vi "SetColorState.vi"(8 "error in (no error)":errorcluster, 10 "ColorStateIn":T1, 11 "Boolean in":refnum<vi>) -> (0 "error out":errorcluster, 2 "ColorStateOut":T1)   [LabVIEW 2016]
uses:
  controls/ColorStates.ctl
  controls/RT-Variables.lvlib
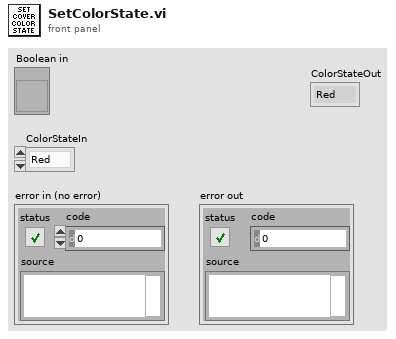
[diagram p1: front panel]
types:
  T1 = typedef "RT-Variables.lvlib/ColorStates.ctl" = enum16{"Red", "Yellow", "Green"}
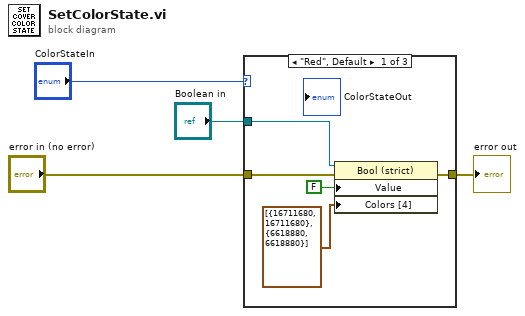
[diagram p0: block diagram]
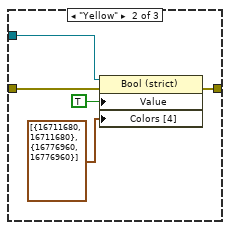
[diagram p2: hidden frame]
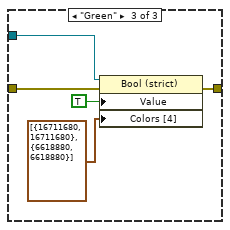
[diagram p3: hidden frame]
diagram:
  n1 = case shown="\"Red\", Default" "ColorStateIn" {
    tunnel: "Boolean in" -> [w7 w12 w17]
    tunnel: "error in (no error)" -> [w6 w11 w15]
    tunnel: [w5 w10 w16] -> w4
    frame "Red", Default {
      n2 = property on="Property Node" class="Bool (strict)"(reference=w7, error in=w6, "Value"=FALSE, "Colors [4]"=cluster{u32, u32}[] [{16711680, 16711680}, {6618880, 6618880}]) -> (error out=w5:errorcluster)  [unwired: 1 out]
    }
    frame "Yellow" {
      n3 = property on="Property Node" class="Bool (strict)"(reference=w12, error in=w11, "Value"=TRUE, "Colors [4]"=cluster{u32, u32}[] [{16711680, 16711680}, {16776960, 16776960}]) -> (error out=w10:errorcluster)  [unwired: 1 out]
    }
    frame "Green" {
      n4 = property on="Property Node" class="Bool (strict)"(reference=w17, error in=w15, "Value"=TRUE, "Colors [4]"=cluster{u32, u32}[] [{16711680, 16711680}, {6618880, 6618880}]) -> (error out=w16:errorcluster)  [unwired: 1 out]
    }
  }
  "error out" <- w4
